vi "MakeExample.vi"(8 "error in (no error)":errorcluster, 9 "TriggerRefractoryPeriod (Frames)":i32, 10 "StimulusObject Parameters":variant, 11 "JustHeadRails in":refnum<class "JustHeadRails.lvclass">) -> (0 "error out":errorcluster, 3 "JustHeadRails out":refnum<class "JustHeadRails.lvclass">)   [LabVIEW 2019, in "JustHeadRails.lvclass"]
uses:
  JustHeadRails.lvclass
  JustTailRailsClass/JustTailRailsInputCluster.ctl
  JustHeadRails.lvclass/JustHeadRails.ctl
  ParametersGlobal.vi
  StimulusObject.lvclass
  JustTailRails.lvclass
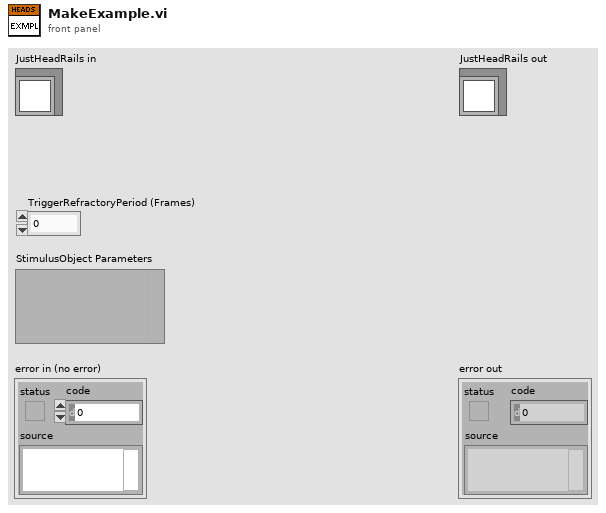
[diagram p1: front panel]
types:
  T1 = typedef "JustTailRails.lvclass/JustTailRailsInputCluster.ctl" = cluster{"Constant Intensity (uW/mm^2, negative is blue)":sgl, "dot radius (mm)":sgl, "Intensities (uW/mm^2, negative is blue)":sgl[], "Durations (s)":sgl[], "Inter trigger interval (s)":dbl}
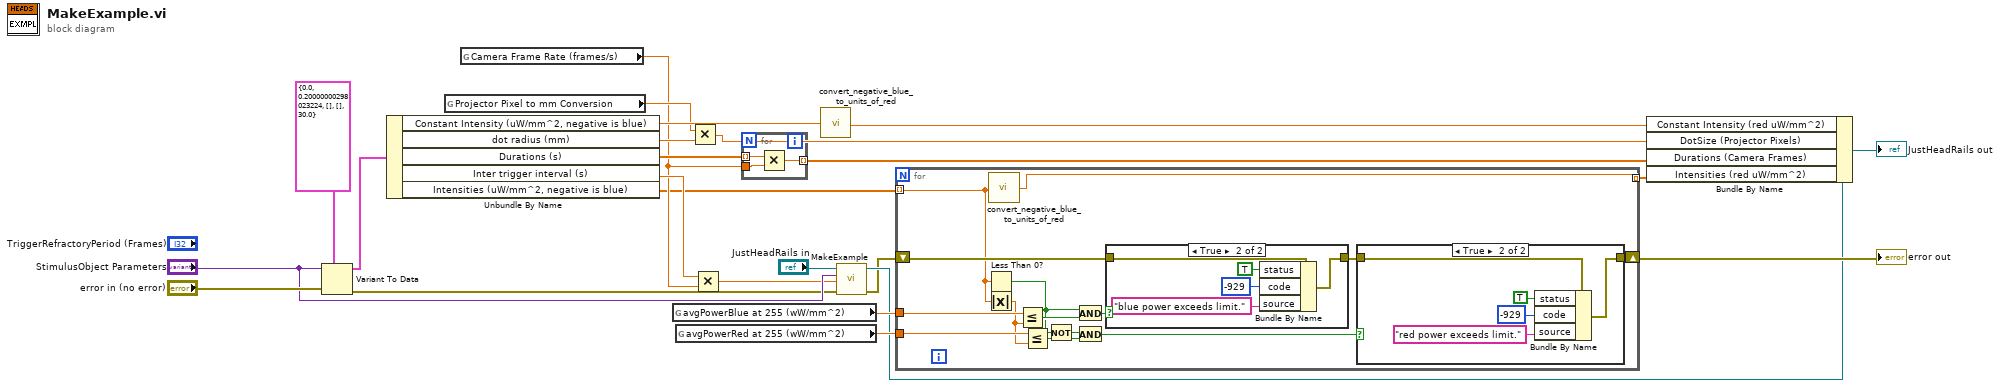
[diagram p0: block diagram]
diagram:
  n1 = Variant To Data(error in="error in (no error)", type=T1 {"Constant Intensity (uW/mm^2, negative is blue)"=0.0, "dot radius (mm)"=0.2, "Intensities (uW/mm^2, negative is blue)"=[], "Durations (s)"=[], "Inter trigger interval (s)"=30.0} ("JustHeadsRailsInputCluster"), Variant="StimulusObject Parameters") -> (data=w24:T1, error out=w3:errorcluster)
  n2 = Unbundle By Name(w24) -> ("Constant Intensity (uW/mm^2, negative is blue)"=w22:sgl, "dot radius (mm)"=w20:sgl, "Durations (s)"=w17:sgl[], "Inter trigger interval (s)"=w23:dbl, "Intensities (uW/mm^2, negative is blue)"=w14:sgl[])
  n3 = global read "ParametersGlobal.vi" "Projector Pixel to mm Conversion"() -> (w19:sgl)
  n4 = global read "ParametersGlobal.vi" "Camera Frame Rate (frames/s)"() -> (w16:sgl)
  n5 = global read "ParametersGlobal.vi" "avgPowerBlue at 255 (wW/mm^2)"() -> (w13:sgl)
  n6 = global read "ParametersGlobal.vi" "avgPowerRed at 255 (wW/mm^2)"() -> (w12:sgl)
  n7 = Multiply(x=w19, y=w20) -> (x*y=w18:sgl)
  n8 = Multiply(x=w23, y=w16) -> (x*y=w4:dbl)
  n9 = for {
    tunnel: w17 -> [w27] mode=indexing
    tunnel: w16 -> [w26]
    tunnel: [w25] -> w15 mode=indexing
    n10 = Multiply(x=w27, y=w26) -> (x*y=w25:sgl)
  }
  n11 = call "convert_negative_blue_to_units_of_red.vi"("Intensity in units of red (positive) and blue (negative)"=w22) -> ("Intensity in units of red (positive and negative)"=w21:sgl)
  n12 = call-parent "MakeExample.vi"("error in (no error)"=w3, "TriggerRefractoryPeriod (Frames)"=w4, "StimulusObject Parameters"="StimulusObject Parameters", "StimulusObject in"="JustHeadRails in") -> ("error out"=w1:errorcluster, "StimulusObject out"=w2:refnum<class "JustHeadRails.lvclass">)  [unwired: 6 in]
  n13 = for {
    tunnel: w14 -> [w35] mode=indexing
    shift-right: [w39] -> w8
    shift-left: w1 -> [w40]
    tunnel: w13 -> [w38]
    tunnel: w12 -> [w37]
    tunnel: [w36] -> w11 mode=indexing
    n14 = Less Than 0?(x=w35) -> (x < 0?=w28:bool)
    n15 = Absolute Value(x=w35) -> (abs(x)=w34:sgl)
    n16 = call "convert_negative_blue_to_units_of_red.vi"("Intensity in units of red (positive) and blue (negative)"=w35) -> ("Intensity in units of red (positive and negative)"=w36:sgl)
    n17 = Less Or Equal?(x=w38, y=w34) -> (x <= y?=w33:bool)
    n18 = Less Or Equal?(x=w37, y=w34) -> (x <= y?=w30:bool)
    n19 = Not(x=w28) -> (.not. x?=w29:bool)
    n20 = And(x=w28, y=w33) -> (x .and. y?=w32:bool)
    n21 = And(x=w29, y=w30) -> (x .and. y?=w31:bool)
    n22 = case shown="True" w32 {
      tunnel: w40 -> [w48 w53]
      tunnel: [w48 w52] -> w41
      frame False {
      }
      frame True {
        n23 = Bundle By Name(cluster=w53, "status"=TRUE, "code"=-929, "source"="blue power exceeds limit.") -> (w52:errorcluster)
      }
    }
    n24 = case shown="True" w31 {
      tunnel: w41 -> [w42 w47]
      tunnel: [w42 w46] -> w39
      frame False {
      }
      frame True {
        n25 = Bundle By Name(cluster=w47, "status"=TRUE, "code"=-929, "source"="red power exceeds limit.") -> (w46:errorcluster)
      }
    }
  }
  "error out" <- w8
  n26 = Bundle By Name(cluster=w2, "Constant Intensity (red uW/mm^2)"=w21, "DotSize (Projector Pixels)"=w18, "Durations (Camera Frames)"=w15, "Intensities (red uW/mm^2)"=w11) -> (→"JustHeadRails out":refnum<class "JustHeadRails.lvclass">)
